vi "ESP301_Home.vi"(8 "mode":i32=2, 9 "homePresetPosition":dbl, 10 "axisNumber":i32=1, 11 "COM_PORT":string="COM12") -> ()   [LabVIEW 2019]
uses:
  Newport.ESP301.CommandInterface
panel:
  out "errstring":string
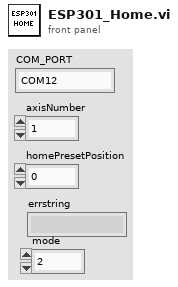
[diagram p1: front panel]
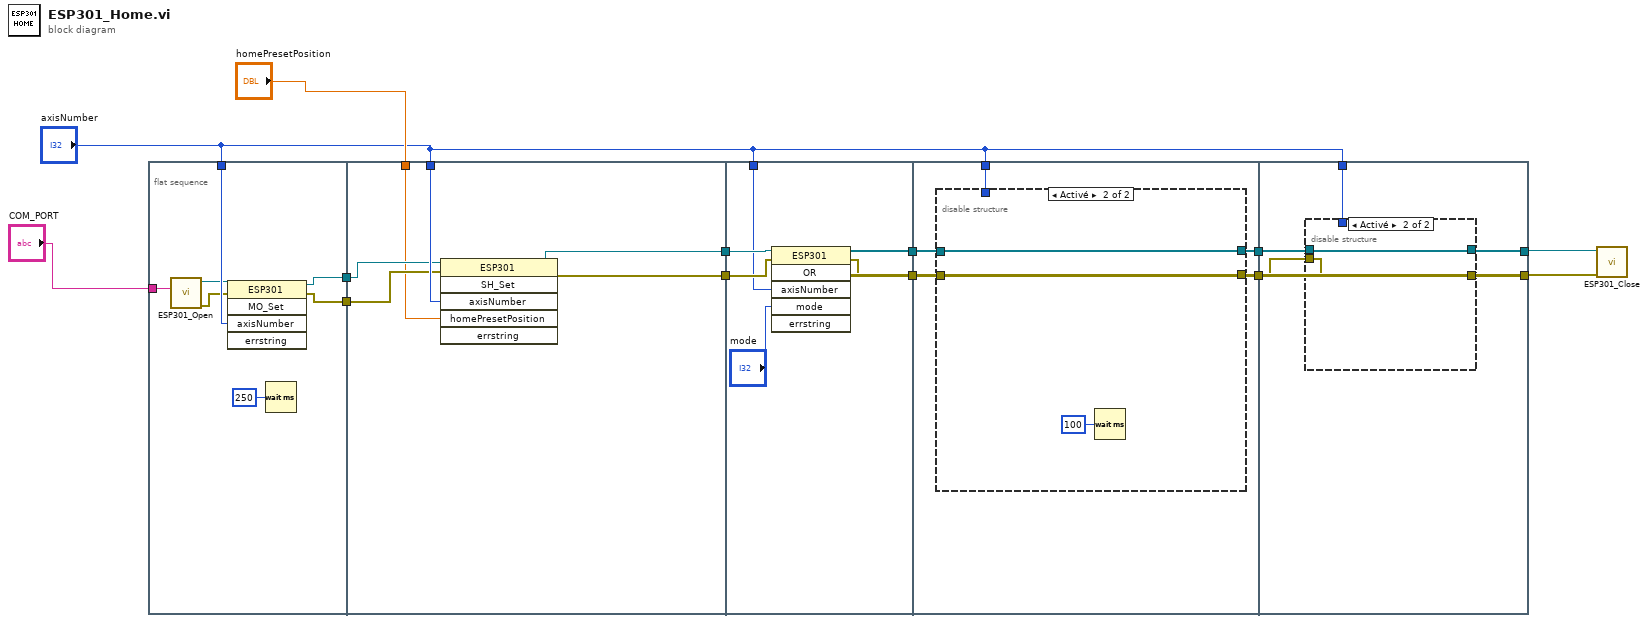
[diagram p0: block diagram]
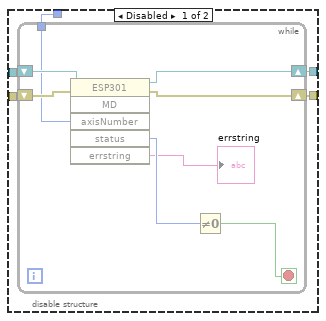
[diagram p2: hidden frame]
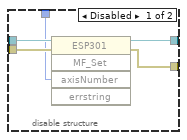
[diagram p3: hidden frame]
diagram:
  n1 = flat-sequence {
    tunnel: [w15] -> w11
    tunnel: [w16] -> w10
    tunnel: "COM_PORT" -> [w20]
    tunnel: "axisNumber" -> [w19]
    tunnel: "axisNumber" -> [w26]
    tunnel: w11 -> [w23]
    tunnel: w10 -> [w22]
    tunnel: [w25] -> w5
    tunnel: [w24] -> w3
    tunnel: "homePresetPosition" -> [w21]
    tunnel: w5 -> [w32]
    tunnel: [w31] -> w4
    tunnel: w3 -> [w29]
    tunnel: [w30] -> w2
    tunnel: "axisNumber" -> [w28]
    tunnel: w4 -> [w36]
    tunnel: w2 -> [w35]
    tunnel: [w34] -> w8
    tunnel: [w33] -> w7
    tunnel: "axisNumber" -> [w37]
    tunnel: [w55] -> w12
    tunnel: [w56] -> w13
    tunnel: w8 -> [w58]
    tunnel: w7 -> [w57]
    tunnel: "axisNumber" -> [w54]
    frame #0 {
      n2 = call "ESP301_Open.vi"("strDeviceKey"=w20) -> ("sortie d'erreur"=w17:errorcluster, "référence en sortie"=w18:refnum<k24>)  [unwired: 9 in]
      n3 = invoke on="Nœud de méthode" class="ESP301" method="MO_Set"(reference=w18, error in=w17, "axisNumber"=w19) -> (reference out=w16:refnum<k24>, error out=w15:errorcluster)  [unwired: 2 in, 3 out]
      n4 = Wait (ms)(milliseconds to wait=u32 250 ("attente (ms)")) -> ()  [unwired: 1 out]
    }
    frame #1 {
      n5 = invoke on="Nœud de méthode" class="ESP301" method="SH_Set"(reference=w22, error in=w23, "axisNumber"=w26, "homePresetPosition"=w21) -> (reference out=w25:refnum<k24>, error out=w24:errorcluster)  [unwired: 2 in, 4 out]
    }
    frame #2 {
      n6 = invoke on="Nœud de méthode" class="ESP301" method="OR"(reference=w32, error in=w29, "axisNumber"=w28, "mode"="mode") -> (reference out=w31:refnum<k24>, error out=w30:errorcluster)  [unwired: 2 in, 4 out]
    }
    frame #3 {
      n7 = disable-structure shown="Activé" {
        disable-tunnel: w37 -> [w42 _]
        disable-tunnel: w36 -> [w41 w53]
        disable-tunnel: w35 -> [w40 w52]
        disable-tunnel: [w39 w53] -> w34
        disable-tunnel: [w38 w52] -> w33
        frame Disabled {
          n8 = while {
            tunnel: w42 -> [w48]
            shift-right: [w47] -> w39
            shift-left: w41 -> [w50]
            shift-right: [w46] -> w38
            shift-left: w40 -> [w49]
            stop <- w45 stop-if-true
            n9 = invoke on="Nœud de méthode" class="ESP301" method="MD"(reference=w50, error in=w49, "axisNumber"=w48) -> (reference out=w47:refnum<k24>, error out=w46:errorcluster, "status"=w44:i32, "errstring"=→"errstring":string)  [unwired: 3 in, 2 out]
            n10 = Not Equal To 0?(x=w44) -> (x != 0?=w45:bool)
          }
        }
        frame Enabled {
          n11 = Wait (ms)(milliseconds to wait=u32 100 ("attente (ms)")) -> ()  [unwired: 1 out]
        }
      }
    }
    frame #4 {
      n12 = disable-structure shown="Activé" {
        disable-tunnel: w58 -> [w63 w65]
        disable-tunnel: w57 -> [w62 w64]
        disable-tunnel: [w61 w65] -> w56
        disable-tunnel: [w60 w64] -> w55
        disable-tunnel: w54 -> [w59 _]
        frame Disabled {
          n13 = invoke on="Nœud de méthode" class="ESP301" method="MF_Set"(reference=w63, error in=w62, "axisNumber"=w59) -> (reference out=w61:refnum<k24>, error out=w60:errorcluster)  [unwired: 2 in, 3 out]
        }
        frame Enabled {
        }
      }
    }
  }
  n14 = call "ESP301_Close.vi"("entrée d'erreur (pas d'erreur)"=w12, "référence"=w13) -> ()  [unwired: 9 in, 1 out]
